vi "Read Network Excel.vi"(8 "error in (no error)":errorcluster caption="错误输入（无错误）", 10 "T/Y":bool, 11 "Base Path":path) -> (0 "error out":errorcluster caption="错误输出", 3 "2DA_Str":string[][](array[string]))   [LabVIEW 2014]
uses:
  <vilib>/Utility/file.llb/Read Delimited Spreadsheet (string).vi
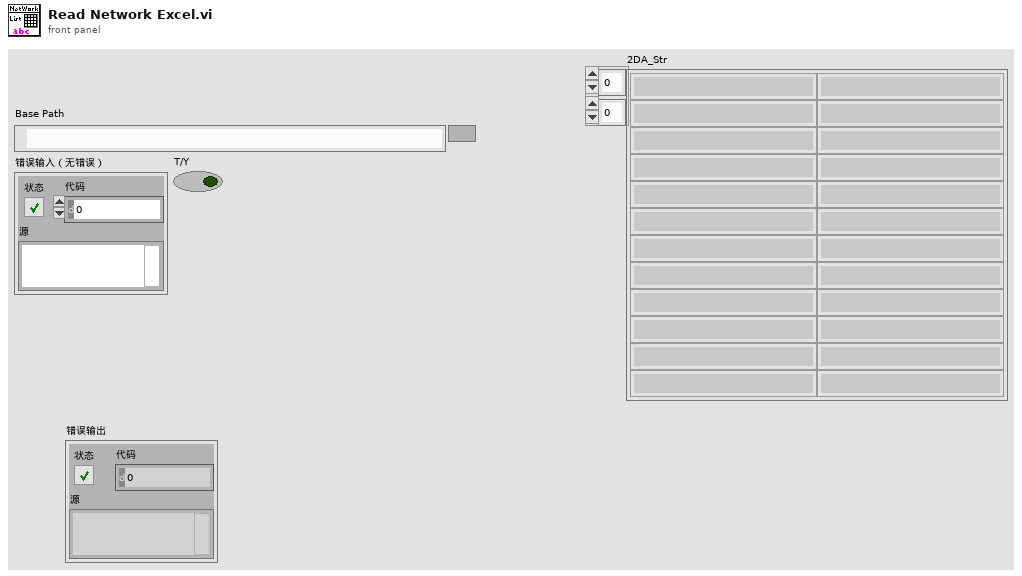
[diagram p1: front panel]
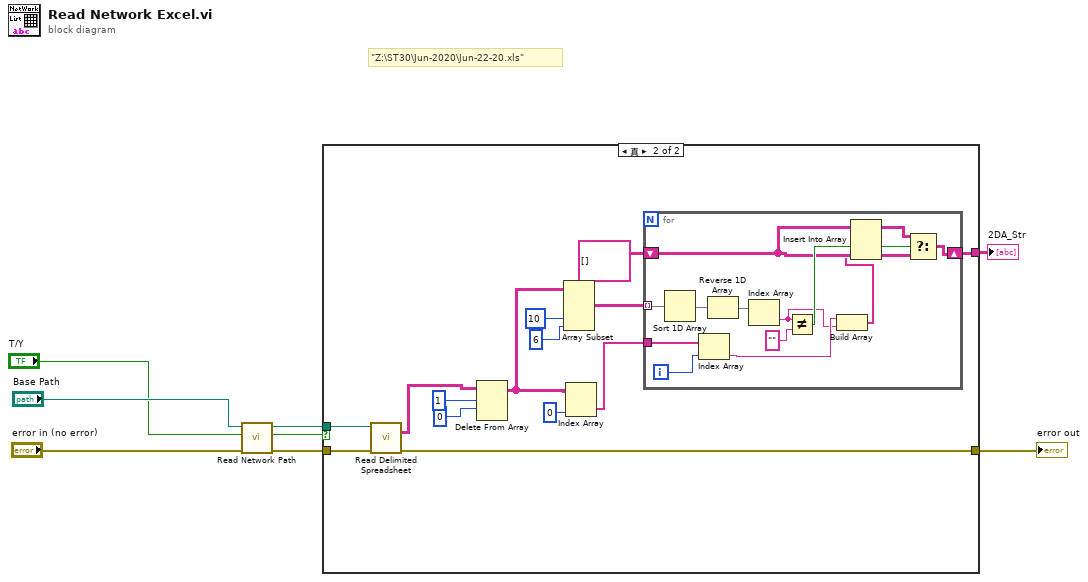
[diagram p0: block diagram]
diagram:
  # "\"Z:\\ST30\\Jun-2020\\Jun-22-20.xls\""
  n1 = call "Read Network Path.vi"("error in (no error)"="error in (no error)", "T/Y"="T/Y", "Base Path"="Base Path") -> ("error out"=w7:errorcluster, "file or folder exists?"=w2:bool, "appended path"=w3:path)  [unwired: 6 in]
  n2 = case shown="真" w2 {
    tunnel: [_ w13] -> w8
    tunnel: w7 -> [w9 w12]
    tunnel: w3 -> [_ w11]
    tunnel: [w9 w10] -> w1
    frame False {
    }
    frame True {
      n3 = call-poly <vilib>:"Read Delimited Spreadsheet.vi"("file path (dialog if empty)"=w11, "error in (no error)"=w12) -> ("all rows"=w23:string[][], "error out"=w10:errorcluster)  [unwired: 8 in, 4 out]
      n4 = Delete From Array(array=w23, length=1 ("长度"), index (row)=0 ("禁用的索引 (列)")) -> (array with subset deleted=w17:string[][])  [unwired: 1 in, 1 out]
      n5 = Array Subset(array=w17, index (col)=10 ("索引"), length (col)=6 ("长度")) -> (w16:string[][])  [unwired: 2 in]
      n6 = Index Array(array=w17, index (col)=0 ("禁用的索引 (列)")) -> (element=w14:string[])  [unwired: 1 in]
      n7 = for {
        tunnel: w16 -> [w34] mode=indexing
        tunnel: w14 -> [w33]
        shift-right: [w29] -> w13
        shift-left: string[][] [] -> [w26]
        i -> [w32]
        n8 = Sort 1D Array(array=w34) -> (sorted array=w36:string[])
        n9 = Index Array(array=w33, index=w32) -> (element=w28:string)
        n10 = Reverse 1D Array(array=w36) -> (reversed array=w35:string[])
        n11 = Index Array(array=w35) -> (element=w27:string)  [unwired: 1 in]
        n12 = Not Equal?(x=w27, y="") -> (x != y?=w30:bool)
        n13 = Build Array(w28, w27) -> (w24:string[])
        n14 = Insert Into Array(array=w26, new element=w24) -> (w25:string[][])  [unwired: 2 in]
        n15 = Select(t=w25, s=w30, f=w26) -> (s? t:f=w29:string[][])
      }
    }
  }
  "2DA_Str" <- w8
  "error out" <- w1
